vi "CCT.vi"(0 "System no.":i32=1 min=1 step=1, 2 "Command type":i32=2, 5 "error in":errorcluster) -> (19 "error out":errorcluster)   [LabVIEW 2026]
doc: "This VI sets the command type (e.g. ASCII or binary) of the controller. \n\nE-761: Command type can be 1 (ASCII) or 2 (binary). Note: After power up the controller communicates via ASCII protocol."
panel:
  # "This vi sets the command type (e.g. ASCII or binary) of the con-\ntroller. See VI description for available types."
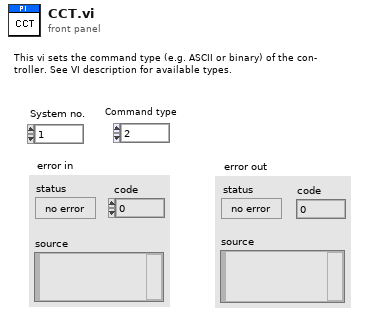
[diagram p1: front panel]
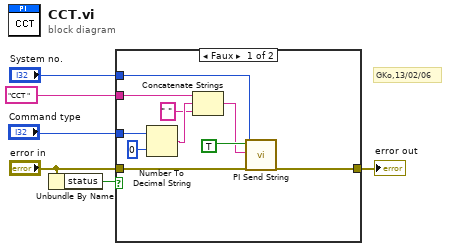
[diagram p0: block diagram]
diagram:
  # "GKo,13/02/06"
  n1 = Unbundle By Name("error in") -> ("status"=w2:bool)
  n2 = case shown="Faux" w2 {
    tunnel: [w7 w17] -> w6
    tunnel: "CCT " -> [w16 _]
    tunnel: "System no." -> [w14 _]
    tunnel: "error in" -> [w12 w17]
    tunnel: "Command type" -> [w11 _]
    frame False {
      n3 = Number To Decimal String(number=w11, width (-)=i16 0) -> (decimal integer string=w9:string)
      n4 = Concatenate Strings(w16, w9, " " ("Substring")) -> (w13:string)
      n5 = call "PI Send String.vi"("System no."=w14, "String to send"=w13, "Attach termination char.?"=TRUE ("Attach Linefeed?"), "error in"=w12) -> ("error out"=w7:errorcluster)  [unwired: 15 out]
    }
    frame True {
    }
  }
  "error out" <- w6
